vi "ElevatorFloorSendCmd.vi"(8 "error in (no error)":errorcluster) -> (0 "error out":errorcluster)   [LabVIEW 2023]
doc: "Sends a boolean command to the boolean receive called \"Floor\" (in ElevatorExecuteLogic.vi) to set the Elevator to Floor pickup height\n\nInputs:\n--error in\nOuputs:\n--error out"
uses:
  <vilib>/Rock Robotics/WPI/ThirdParty/JAS_Junk/TrajLib/Trajectory_Library.lvlib
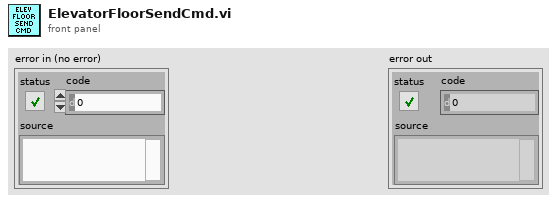
[diagram p1: front panel]
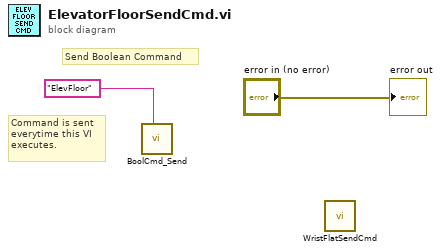
[diagram p0: block diagram]
diagram:
  # "Command is sent\neverytime this VI\nexecutes."
  # "Send Boolean Command"
  n1 = call <vilib>:"BoolCmd_Send.vi"("Command Name"="ElevFloor") -> ()  [unwired: 10 in, 1 out]
  n2 = call "WristFlatSendCmd.vi"() -> ()  [unwired: 11 in, 1 out]
  "error out" <- "error in (no error)"
